vi "Stop.vi"(8 "error in (no error)":errorcluster, 10 "Emergency Stop (F)":bool, 11 "Actor API in":refnum<class "Actor API.lvclass">) -> (0 "error out":errorcluster, 3 "Actor API out":refnum<class "Actor API.lvclass">)   [LabVIEW 2020, in "Artifex.lvlib" / "Actor API.lvclass"]
uses:
  Actor API.lvclass
  Priority.ctl
  Artifex.lvlib
  Stop Msg/Stop Msg.lvclass
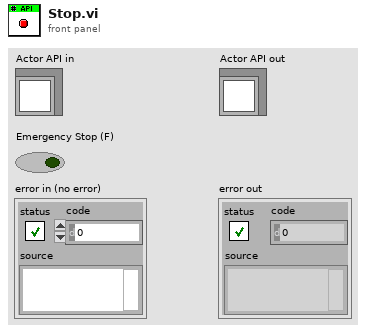
[diagram p1: front panel]
types:
  T1 = typedef "Artifex.lvlib/Priority.ctl" = enum16{"Low", "Normal", "High"}
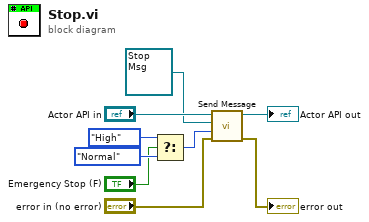
[diagram p0: block diagram]
diagram:
  n1 = Select(t=Priority."High" ("Priority"), s="Emergency Stop (F)", f=Priority."Normal" ("Priority")) -> (s? t:f=w3:T1)
  n2 = call "Send Message.vi"("error in (no error)"="error in (no error)", "Priority (Normal)"=w3, "Message"=refnum<class "Stop Msg.lvclass"> refnum ("Artifex.lvlib:Stop Msg.lvclass"), "Actor API in"="Actor API in") -> ("error out"=→"error out":errorcluster, "Actor API out"=→"Actor API out":refnum<class "Actor API.lvclass">)  [unwired: 6 in]
